vi "Zadanie Testowe.vi"() -> ()   [LabVIEW 2015]
panel:
  out "Wynik":dbl
  in  "x":dbl
  in  "Parametr a0":dbl
  in  "Parametr a1":dbl
  in  "Parametr a2":dbl
  in  "Parametr a3":dbl
  # "Wyliczanie równania a3x^3+a2x^2+a1x+a0"
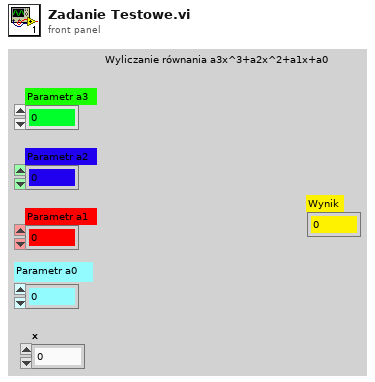
[diagram p1: front panel]
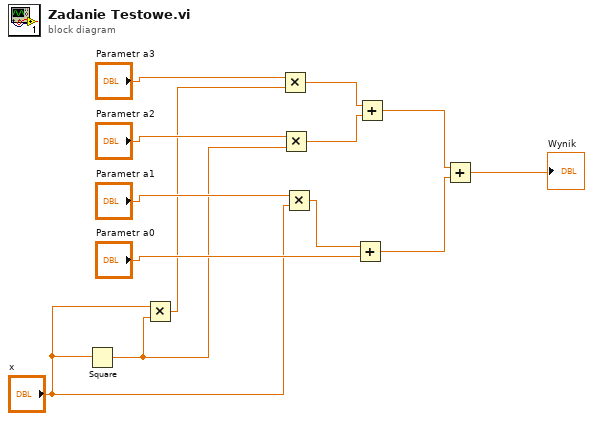
[diagram p0: block diagram]
diagram:
  n1 = Square(x="x") -> (x^2=w2:dbl)
  n2 = Multiply(x="x", y=w2) -> (x*y=w1:dbl)
  n3 = Multiply(x="Parametr a3", y=w1) -> (x*y=w7:dbl)
  n4 = Multiply(x="Parametr a2", y=w2) -> (x*y=w8:dbl)
  n5 = Multiply(x="Parametr a1", y="x") -> (x*y=w9:dbl)
  n6 = Add(x=w9, y="Parametr a0") -> (x+y=w5:dbl)
  n7 = Add(x=w7, y=w8) -> (x+y=w6:dbl)
  n8 = Add(x=w6, y=w5) -> (x+y=→"Wynik":dbl)
